vi "Postion Finder.vi"(5 "derivitave":i8, 7 "Max profiles":T1, 10 "TimeSegments":T2, 11 "time":dbl) -> (3 "Motion Profiler Setpoint":dbl)   [LabVIEW 2014]
uses:
  TimeSegments.ctl
  TimeSegment.ctl
  Max profiles.ctl
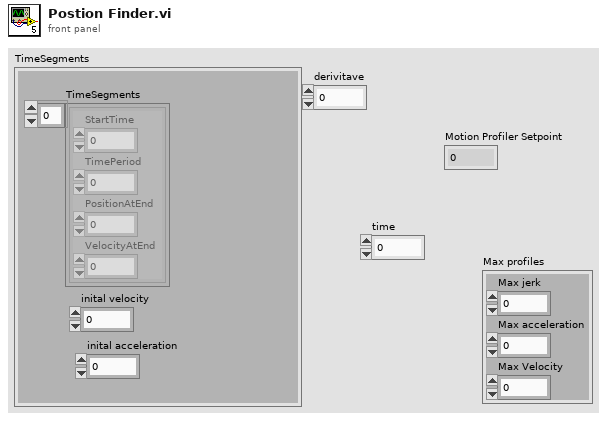
[diagram p1: front panel]
types:
  T1 = typedef "Max profiles.ctl" = cluster{"Max jerk":dbl, "Max acceleration":dbl, "Max Velocity":dbl}
  T2 = typedef "TimeSegments.ctl" = cluster{"TimeSegments":T3[], "inital velocity":dbl, "inital acceleration":dbl}
  T3 = typedef "TimeSegment.ctl" = cluster{"StartTime":dbl, "TimePeriod":dbl, "PositionAtEnd":dbl, "VelocityAtEnd":dbl}
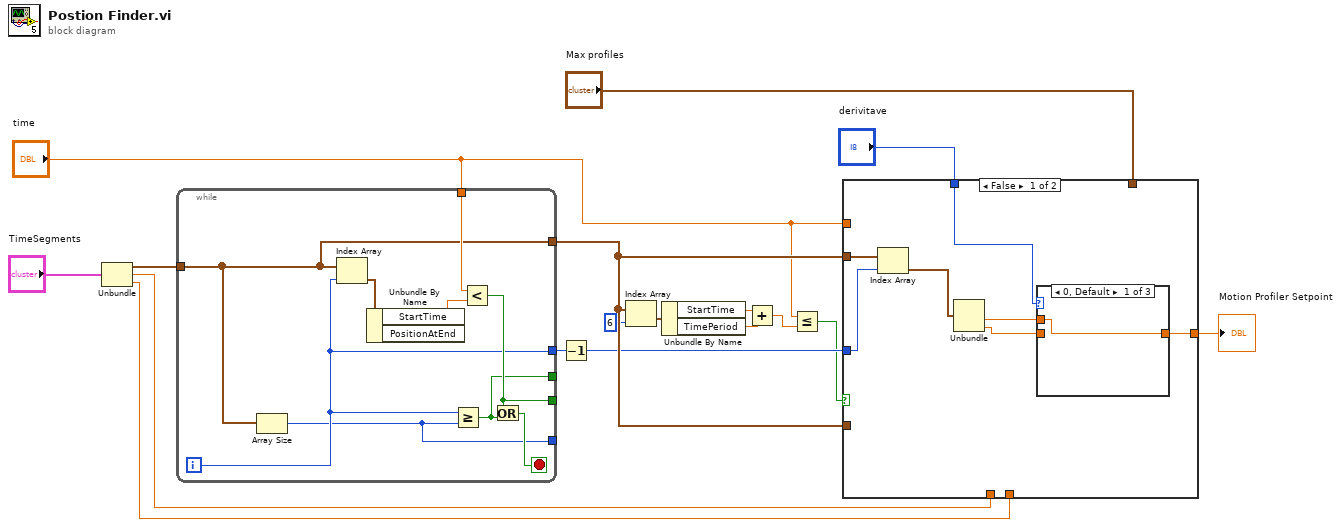
[diagram p0: block diagram]
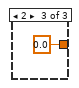
[diagram p3: hidden frame]
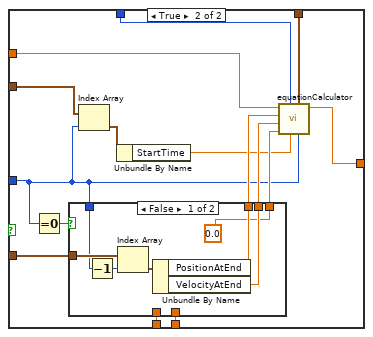
[diagram p4: hidden frame]
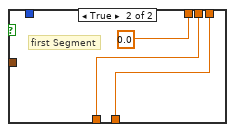
[diagram p5: hidden frame]
diagram:
  n1 = Unbundle("TimeSegments") -> ("TimeSegments"=w14:T3[], "inital velocity"=w13:dbl, "inital acceleration"=w12:dbl)
  n2 = while {
    tunnel: "time" -> [w25]
    tunnel: [w24] -> _
    tunnel: [w22] -> w10
    tunnel: [w20] -> w9
    tunnel: w14 -> [w20]
    tunnel: [w19] -> _
    tunnel: [w18] -> _
    i -> [w22]
    stop <- w26 stop-if-true
    n3 = Array Size(array=w20) -> (size(s)=w18:i32)
    n4 = Index Array(array=w20, index=w22) -> (element=w23:T3)
    n5 = Unbundle By Name(w23) -> ("StartTime"=w21:dbl)  [unwired: 1 out]
    n6 = Greater Or Equal?(x=w22, y=w18) -> (x >= y?=w19:bool)
    n7 = Less?(x=w25, y=w21) -> (x < y?=w24:bool)
    n8 = Or(x=w24, y=w19) -> (x .or. y?=w26:bool)
  }
  n9 = Decrement(x=w10) -> (x-1=w8:i32)
  n10 = Index Array(array=w9, index=6) -> (element=w7:T3)
  n11 = Unbundle By Name(w7) -> ("StartTime"=w6:dbl, "TimePeriod"=w5:dbl)
  n12 = Add(x=w6, y=w5) -> (x+y=w3:dbl)
  n13 = Less Or Equal?(x="time", y=w3) -> (x <= y?=w2:bool)
  n14 = case shown="False" w2 {
    tunnel: w8 -> [w32 w37]
    tunnel: [w28 w51] -> w17
    tunnel: "Max profiles" -> [_ w50]
    tunnel: "time" -> [_ w49]
    tunnel: w9 -> [_ w47]
    tunnel: w13 -> [_ w44]
    tunnel: w12 -> [_ w43]
    tunnel: "derivitave" -> [w30 w41]
    tunnel: w9 -> [w33 w40]
    frame False {
      n15 = Index Array(array=w33, index=w32) -> (element=w31:T3)
      n16 = Unbundle(w31) -> ("PositionAtEnd"=w29:dbl, "VelocityAtEnd"=w27:dbl)  [unwired: 2 out]
      n17 = case shown="0, Default" w30 {
        tunnel: w29 -> [w34 _ _]
        tunnel: [w34 w35 0.0 ("VelocityAtEnd")] -> w28
        tunnel: w27 -> [_ w35 _]
        frame 0, Default {
        }
        frame 1 {
        }
        frame 2 {
        }
      }
    }
    frame True {
      n18 = Equal To 0?(x=w37) -> (x = 0?=w48:bool)
      n19 = case shown="False" w48 {
        tunnel: w47 -> [w58 _]
        tunnel: w37 -> [w57 _]
        tunnel: [w54 0.0 ("PositionAtEnd")] -> w46
        tunnel: [w53 w60] -> w45
        tunnel: w44 -> [_ w60]
        tunnel: w43 -> [_ w59]
        tunnel: [0.0 ("inital acceleration") w59] -> w42
        frame False {
          n20 = Decrement(x=w57) -> (x-1=w56:i32)
          n21 = Index Array(array=w58, index=w56) -> (element=w55:T3)
          n22 = Unbundle By Name(w55) -> ("PositionAtEnd"=w54:dbl, "VelocityAtEnd"=w53:dbl)
        }
        frame True {
          # "first Segment"
        }
      }
      n23 = Index Array(array=w40, index=w37) -> (element=w39:T3)
      n24 = Unbundle By Name(w39) -> ("StartTime"=w38:dbl)
      n25 = call "equationCalculator.vi"("Time Segment"=w37, "Max profiles"=w50, "startOfTimePeriod"=w38, "derivitave"=w41, "aInital (only needed for T0)"=w42, "vInital"=w45, "xInital"=w46, "currentTime"=w49) -> ("output variable"=w51:dbl)  [unwired: 3 in]
    }
  }
  "Motion Profiler Setpoint" <- w17
